vi "Sequence.vi"() -> ()   [LabVIEW 2011]
doc: "The Sequence VI acquires a sequence of images and displays the images in an image control using high-level acquisition VIs. A sequence is appropriate for applications in which you want to process multiple images."
uses:
  <vilib>/vision/driver/NI_Vision_Acquisition_Software.lvlib
panel:
  in  "Stop":bool
  in  "Camera Name":refnum<k21> caption="IMAQdx Session"
  out "Image Array":T1[](array[plugin-control])
  in  "Number of Images":i32=5
  # "Overview: Demonstrates how to  acquire a sequence of images and displays them in an array of image controls.\nRequirements: Vision Acquisition Software, IMAQ frame grabber.\nInstructions: \n1. Select the Camera Name\n2. Run the VI."
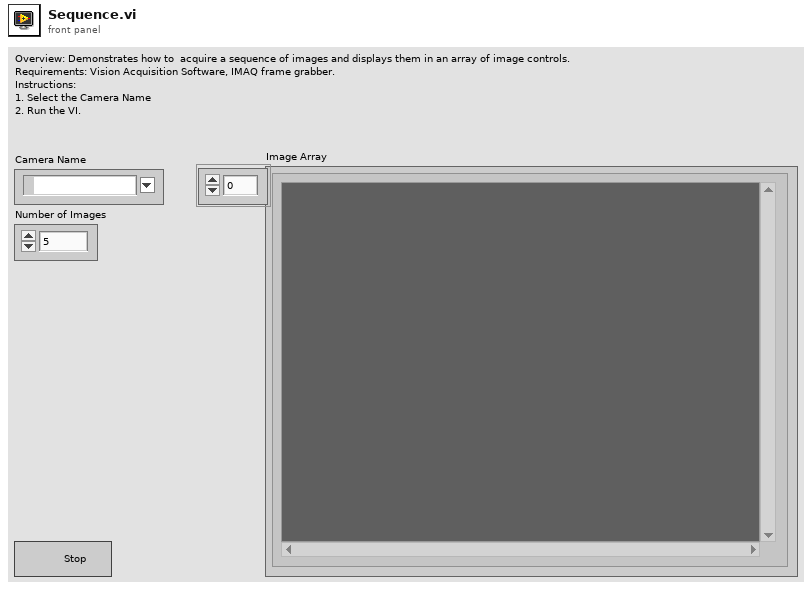
[diagram p1: front panel]
types:
  T1 = typedef "IMAQ Image.ctl" = refnum<image>
  T2 = typedef "IMAQdx.ctl" = refnum<k21>
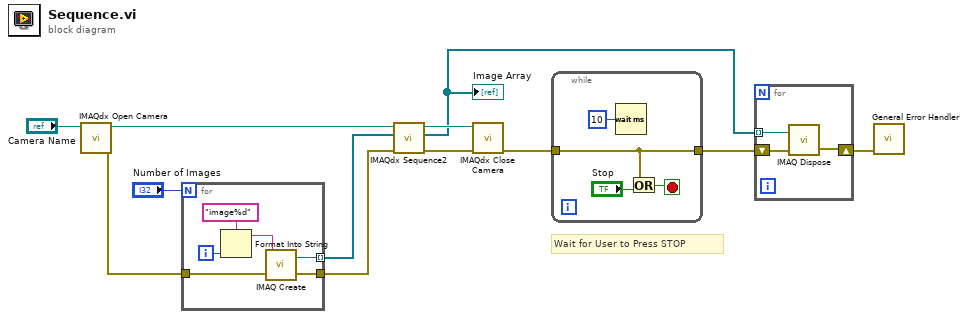
[diagram p0: block diagram]
diagram:
  # "Wait for User to Press STOP"
  n1 = call <vilib>:"IMAQdx Open Camera.vi"("Session In"="Camera Name") -> ("error out"=w11:errorcluster, "Session Out"=w6:T2)  [unwired: 2 in, 7 out]
  n2 = for {
    N: "Number of Images" -> [_]
    tunnel: w11 -> [w18]
    tunnel: [w17] -> w8 mode=indexing
    tunnel: [w16] -> w9
    i -> [w15]
    n3 = Format Into String(format string="image%d" ("Image Name"), w15) -> (resulting string=w14:string)  [unwired: 2 in, 1 out]
    n4 = call "IMAQ Create"("Image Name"=w14, "error in (no error)"=w18) -> ("New Image"=w17:T1, "error out"=w16:errorcluster)  [unwired: 2 in, 1 out]
  }
  n5 = call <vilib>:"IMAQdx Sequence2.vi"("error in"=w9, "Images In"=w8, "Session In"=w6) -> ("error out"=w7:errorcluster, "Images Out"=w2:T1[], "Session Out"=w5:T2)  [unwired: 6 in]
  "Image Array" <- w2
  n6 = call <vilib>:"IMAQdx Close Camera.vi"("error in"=w7, "Session In"=w5) -> ("error out"=w1:errorcluster)  [unwired: 9 out]
  n7 = while {
    tunnel: [w19] -> w4
    tunnel: w1 -> [w19]
    stop <- w20 stop-if-true
    n8 = Wait (ms)(milliseconds to wait=u32 10) -> ()  [unwired: 1 out]
    n9 = Or(x=w19, y="Stop") -> (x .or. y?=w20:bool)
  }
  n10 = for {
    tunnel: w2 -> [w25] mode=indexing
    shift-right: [w23] -> w3
    shift-left: w4 -> [w24]
    n11 = call "IMAQ Dispose"("Image"=w25, "error in (no error)"=w24) -> ("error out"=w23:errorcluster)  [unwired: 1 in, 3 out]
  }
  n12 = call <vilib>:"General Error Handler.vi"("error in (no error)"=w3) -> ()  [unwired: 1 in, 14 out]
